vi "Write On time.vi"(8 "error in (no error)":errorcluster, 10 "On time":timestamp, 11 "SciShutt in":refnum<class "SciShutt.lvclass">) -> (0 "error out":errorcluster, 3 "SciShutt out":refnum<class "SciShutt.lvclass">)   [LabVIEW 2016, in "SciShutt.lvclass"]
uses:
  SciShutt.lvclass
  SciShutt.lvclass/SciShutt.ctl
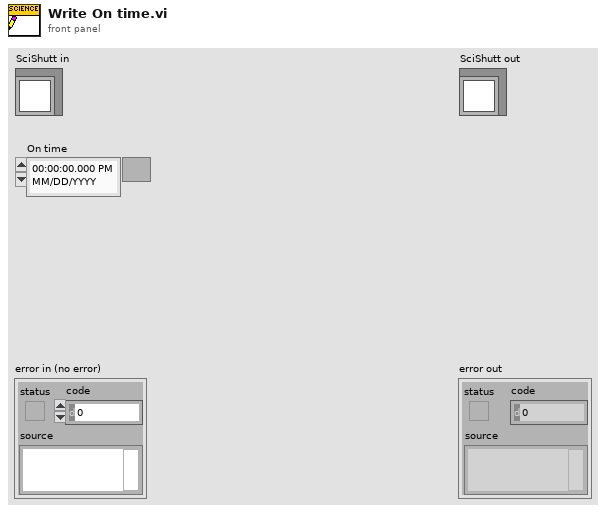
[diagram p1: front panel]
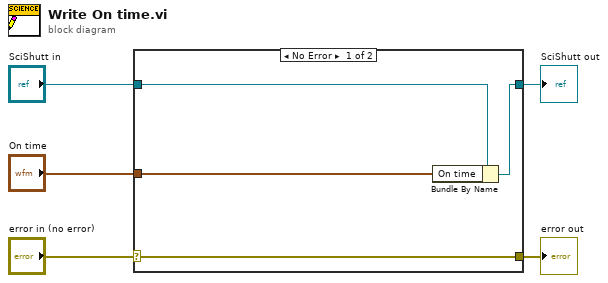
[diagram p0: block diagram]
diagram:
  n1 = case shown="No Error" "error in (no error)" {
    selector: "error in (no error)" -> [w9 w10]
    tunnel: [w9 w10] -> w4
    tunnel: [w7 w11] -> w2
    tunnel: "SciShutt in" -> [w8 w11]
    tunnel: "On time" -> [w6 _]
    frame No Error {
      n2 = Bundle By Name(cluster=w8, "On time"=w6) -> (w7:refnum<class "SciShutt.lvclass">)
    }
    frame Error {
    }
  }
  "error out" <- w4
  "SciShutt out" <- w2
